vi "Match Regular Expression (VI Version).vi"(1 "ignore case? (F)":bool, 2 "multiline? (F)":bool, 3 "return results? (T)":bool=TRUE, 5 "input string":string, 7 "regular expression":string, 9 "offset (0)":i32, 11 "error in":errorcluster) -> (4 "before match":string, 6 "whole match":string, 8 "after match":string, 10 "offset past match":i32, 13 "Capturing goup offsets":cluster{"Start":i32, "After":i32}[](array[cluster]), 14 "Capturing goups":string[](array[string]), 15 "error out":errorcluster)   [LabVIEW 2013]
doc: "Copyright 2018, Carya Automatisering, Wiebe Walstra."
panel:
  # "NOTE:\nThe dll uses string handles. This will sometimes result in unexpected results (empty strings\\crashes) when this VI is run without caller."
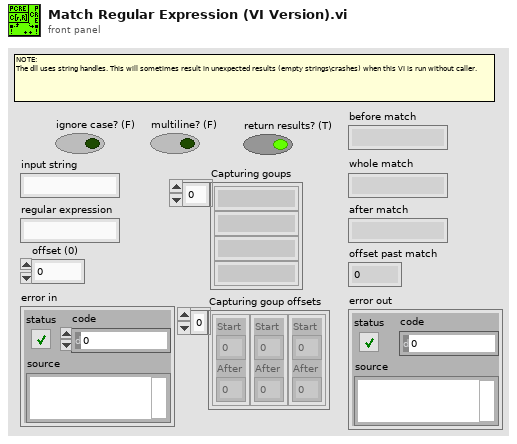
[diagram p1: front panel]
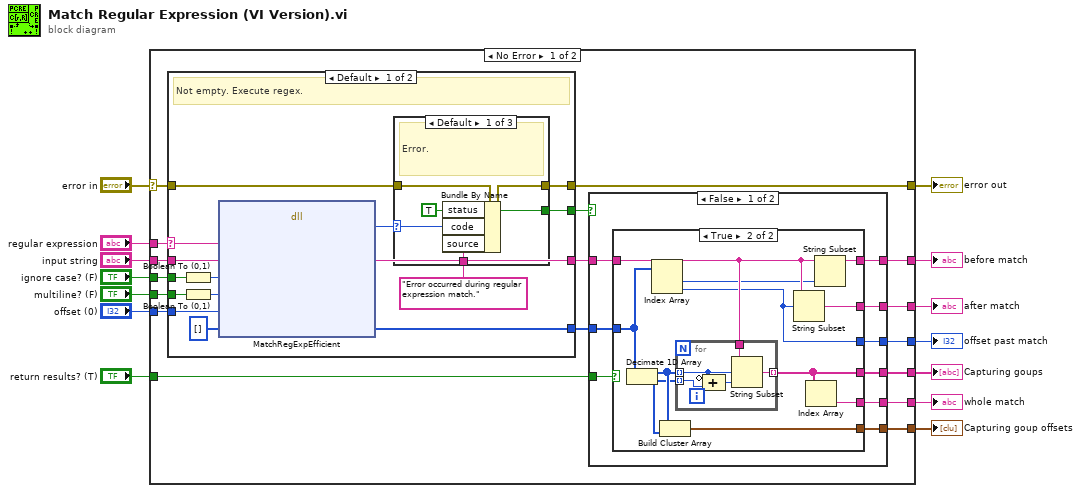
[diagram p0: block diagram]
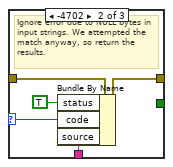
[diagram p2: hidden frame]
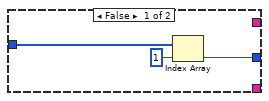
[diagram p5: hidden frame]
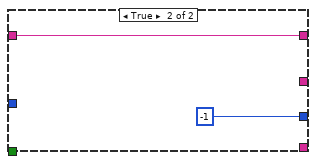
[diagram p6: hidden frame]
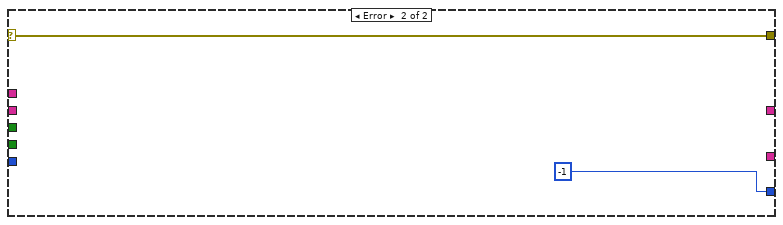
[diagram p7: hidden frame]
diagram:
  n1 = case shown="No Error" "error in" {
    selector: "error in" -> [w20 w89]
    tunnel: [w31 _] -> w3
    tunnel: "input string" -> [w22 _]
    tunnel: [w29 w89] -> w5
    tunnel: [w30 _] -> w13
    tunnel: [w18 -1] -> w6
    tunnel: "multiline? (F)" -> [w23 _]
    tunnel: "ignore case? (F)" -> [w24 _]
    tunnel: "offset (0)" -> [w27 _]
    tunnel: "regular expression" -> [w19 _]
    tunnel: [w26 _] -> w12
    tunnel: [w25 _] -> w14
    tunnel: [w16 _] -> w2
    tunnel: "return results? (T)" -> [w15 _]
    frame No Error {
      n2 = case shown="Default" w19 {
        selector: w19 -> [w37 _]
        tunnel: w24 -> [w41 _]
        tunnel: w23 -> [w45 _]
        tunnel: [w32 _] -> w28
        tunnel: [w44 w57] -> w29
        tunnel: w22 -> [w33 w58]
        tunnel: w27 -> [w40 _]
        tunnel: [w33 w58] -> w21
        tunnel: w20 -> [w34 w57]
        tunnel: [w35 _] -> w17
        frame Default {
          # "Not empty. Execute regex."
          n3 = Boolean To (0,1)(Boolean=w41) -> (0, 1=w43:i16)
          n4 = Boolean To (0,1)(Boolean=w45) -> (0, 1=w42:i16)
          n5 = dll-call lib="LabVIEW" fn="MatchRegExpEfficient"("regexp"=w37, "subject"=w33, "noCase"=w43, "multiline"=w42, "offsetIn"=w40, "offsetsOut"=i32[] [] ("matches")) -> ("return type"=w38:i32, "offsetsOut"=w32:i32[])  [unwired: 8 in, 2 out]
          n6 = case shown="Default" w38 {
            selector: w38 -> [w49 w53 _]
            tunnel: w34 -> [w50 w51 w56]
            tunnel: [w47 w54 w56] -> w44
            tunnel: "Error occurred during regular expression match." ("source") -> [w48 w52 _]
            tunnel: [w46 _ _] -> w35
            frame Default {
              w46 = TRUE ("status")
              # "Error."
              n7 = Bundle By Name(cluster=w50, "status"=w46, "code"=w49, "source"=w48) -> (w47:errorcluster)
            }
            frame -4702 {
              # "Ignore error due to NULL bytes in input strings. We attempted the match anyway, so return the results."
              n8 = Bundle By Name(cluster=w51, "status"=TRUE, "code"=w53, "source"=w52) -> (w54:errorcluster)
            }
            frame 0 {
              # "No error."
            }
          }
        }
        frame "" {
          # "Empty regex. Everything is after match (as \"match pattern\")."
        }
      }
      n9 = case shown="False" w17 {
        tunnel: [w67 _] -> w31
        tunnel: w21 -> [w66 w87]
        tunnel: [w62 _] -> w30
        tunnel: w28 -> [w63 _]
        tunnel: [w64 _] -> w26
        tunnel: [w65 w87] -> w25
        tunnel: [w59 -1] -> w18
        tunnel: [w61 _] -> w16
        tunnel: w15 -> [w60 _]
        frame False {
          n10 = case shown="True" w60 {
            tunnel: [_ w72] -> w67
            tunnel: w66 -> [_ w77]
            tunnel: [_ w76] -> w65
            tunnel: [_ w78] -> w64
            tunnel: w63 -> [w70 w74]
            tunnel: [_ w81] -> w62
            tunnel: [_ w73] -> w61
            tunnel: [w68 w71] -> w59
            frame False {
              n11 = Index Array(array=w70, index=1) -> (element=w68:i32)
            }
            frame True {
              n12 = Decimate 1D Array(w74) -> (w80:i32[], w79:i32[])
              n13 = Index Array(array=w74) -> (element #1=w75:i32, element #2=w71:i32)  [unwired: 2 in]
              n14 = Build Cluster Array(w80, w79) -> (w73:cluster{i32, i32}[])
              n15 = for {
                tunnel: w77 -> [w85]
                tunnel: [w84] -> w72 mode=indexing
                tunnel: w80 -> [w83] mode=indexing
                tunnel: w79 -> [w82] mode=indexing
                n16 = Compound Arithmetic op=ADD(invert w83, w82) -> (w86:i32)
                n17 = String Subset(string=w85, offset (0)=w83, length (rest)=w86) -> (substring=w84:string)
              }
              n18 = String Subset(string=w77, offset (0)=w71) -> (substring=w78:string)  [unwired: 1 in]
              n19 = Index Array(array=w72) -> (element=w81:string)  [unwired: 1 in]
              n20 = String Subset(string=w77, length (rest)=w75) -> (substring=w76:string)  [unwired: 1 in]
            }
          }
        }
        frame True {
        }
      }
    }
    frame Error {
    }
  }
  "before match" <- w14
  "whole match" <- w13
  "after match" <- w12
  "offset past match" <- w6
  "error out" <- w5
  "Capturing goups" <- w3
  "Capturing goup offsets" <- w2
